vi "Log enable.vi"(8 "error in (no error)":errorcluster, 10 "Log":bool, 11 "GUI_Graph in":refnum<class "GUI_Graph.lvclass">) -> (0 "error out":errorcluster, 3 "GUI_Graph out":refnum<class "GUI_Graph.lvclass">)   [LabVIEW 2020, in "GUI_Graph.lvlib" / "GUI_Graph.lvclass"]
uses:
  GUI_Graph.lvclass
  GUI_Graph.lvclass/GUI_Graph.ctl
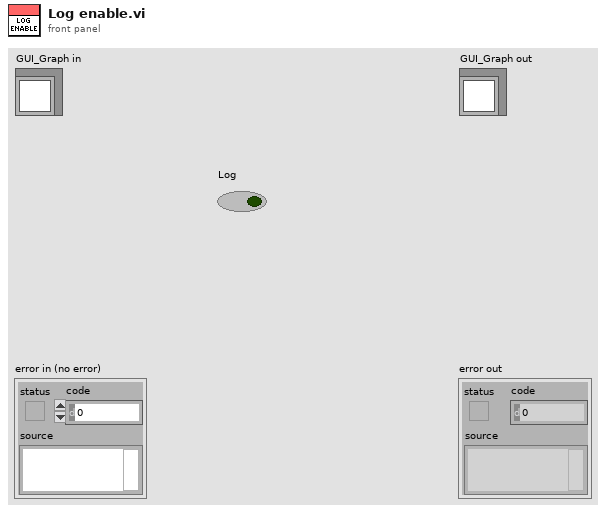
[diagram p1: front panel]
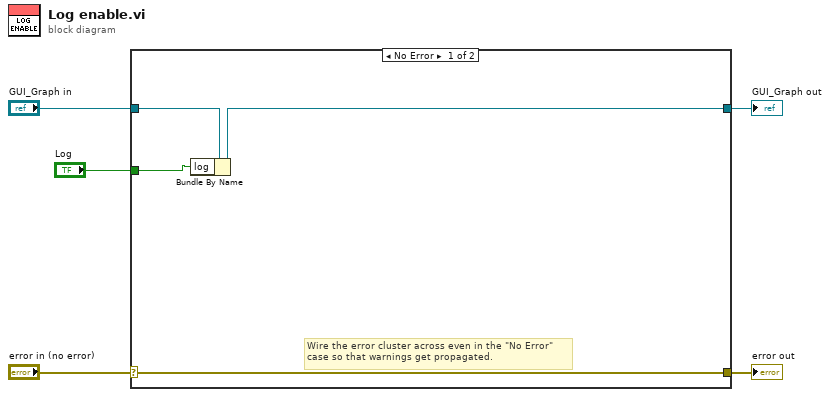
[diagram p0: block diagram]
diagram:
  n1 = case shown="No Error" "error in (no error)" {
    selector: "error in (no error)" -> [w8 w11]
    tunnel: [w8 w11] -> w4
    tunnel: [w7 w10] -> w2
    tunnel: "GUI_Graph in" -> [w9 w10]
    tunnel: "Log" -> [w6 _]
    frame No Error {
      # "Wire the error cluster across even in the \"No Error\"\ncase so that warnings get propagated."
      n2 = Bundle By Name(cluster=w9, "log"=w6) -> (w7:refnum<class "GUI_Graph.lvclass">)
    }
    frame Error {
    }
  }
  "error out" <- w4
  "GUI_Graph out" <- w2
